vi "NewRobotTurningAroundBall.vi"(6 "Target":dbl[](array[numeric]), 7 "Game":refnum<class "Game.lvclass">, 8 "error in (no error)":errorcluster, 9 "Raio":dbl=123.0, 10 "Robot in":refnum<class "Robot.lvclass">, 11 "KickToSkill in":refnum<class "KickToSkill.lvclass">) -> (0 "error out":errorcluster, 1 "Robot out":refnum<class "Robot.lvclass">, 3 "KickToSkill out":refnum<class "KickToSkill.lvclass">)   [LabVIEW 2021, in "KickToSkill.lvclass"]
uses:
  KickToSkill.lvclass
  robotTurningBallStates.ctl
  <vilib>/Analysis/NI_AALPro.lvlib
  <vilib>/Analysis/coordinate.llb/2D Cartesian Coordinate Rotation (Scalar).vi
  Game_class/Game.lvclass
  Robot_class/Robot.lvclass
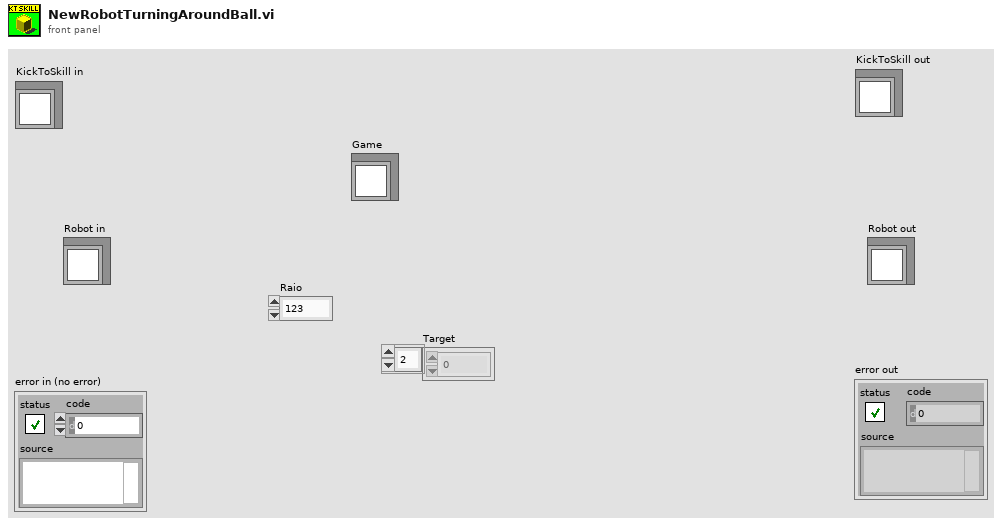
[diagram p1: front panel]
types:
  T1 = typedef "KickToSkill.lvclass/robotTurningBallStates.ctl" = enum16{"go straight to the target", "go to point A", "circulating the ball", "lining up", "shoot"}
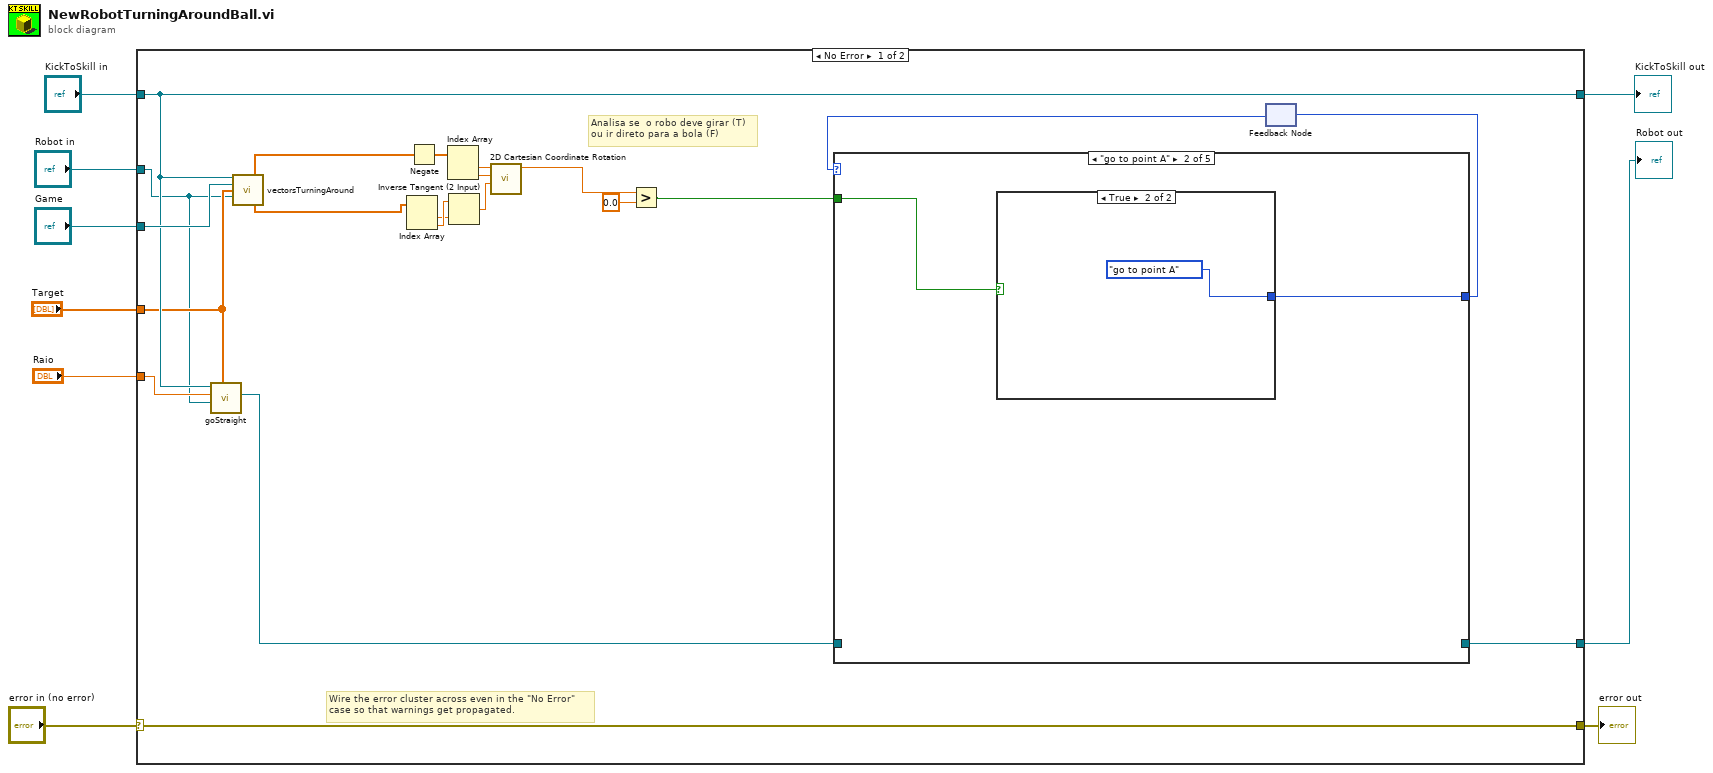
[diagram p0: block diagram]
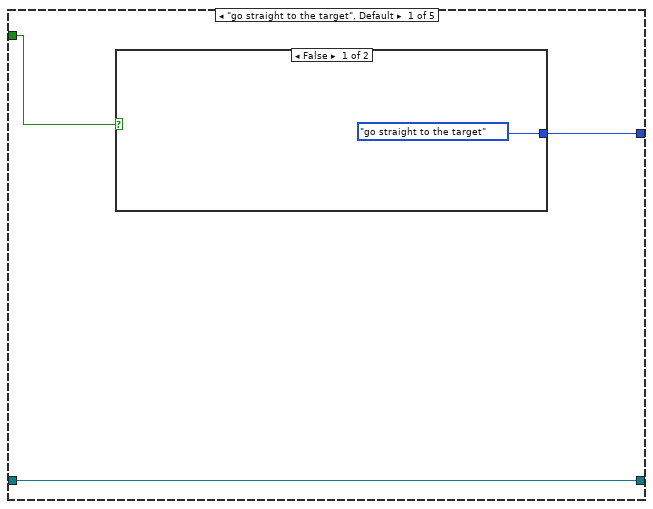
[diagram p2: hidden frame]
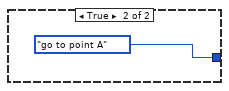
[diagram p3: hidden frame]
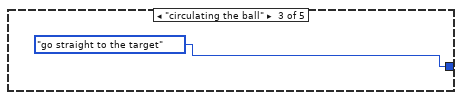
[diagram p5: hidden frame]
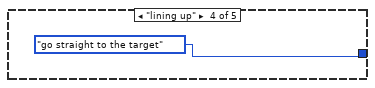
[diagram p6: hidden frame]
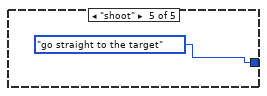
[diagram p7: hidden frame]
diagram:
  n1 = case shown="No Error" "error in (no error)" {
    selector: "error in (no error)" -> [w30 w44]
    tunnel: [w30 w44] -> w8
    tunnel: [w15 w43] -> w6
    tunnel: "KickToSkill in" -> [w15 w43]
    tunnel: "Robot in" -> [w12 w42]
    tunnel: "Target" -> [w14 _]
    tunnel: "Game" -> [w29 _]
    tunnel: "Raio" -> [w13 _]
    tunnel: [w10 w42] -> w1
    frame No Error {
      # "Analisa se  o robo deve girar (T)\nou ir direto para a bola (F)"
      # "Wire the error cluster across even in the \"No Error\"\ncase so that warnings get propagated."
      n2 = call "goStraight.vi"("Target"=w14, "Robot in"=w12, "Raio"=w13, "KickToSkill in"=w15) -> ("Robot out"=w11:refnum<class "Robot.lvclass">)  [unwired: 5 in, 2 out]
      n3 = call "vectorsTurningAround.vi"("KickToSkill in"=w15, "Game"=w29, "Target"=w14, "Robot in"=w12) -> ("Ball - Target"=w20:dbl[], "Robot - Ball"=w19:dbl[])  [unwired: 4 in, 6 out]
      n4 = Index Array(array=w19) -> (element #1=w23:dbl, element #2=w24:dbl)  [unwired: 2 in]
      n5 = Negate(x=w20) -> (-x=w21:dbl[])
      n6 = Index Array(array=w21) -> (element #1=w25:dbl, element #2=w26:dbl)  [unwired: 2 in]
      n7 = Inverse Tangent (2 Input)(1:w23, 2:w24) -> (0:w22:dbl)
      n8 = call-poly <vilib>:"2D Cartesian Coordinate Rotation.vi"("theta"=w22, "y"=w26, "x"=w25) -> ("x out"=w18:dbl)  [unwired: 6 in, 2 out]
      n9 = Greater?(x=w18, y=0.0) -> (0:w16:bool)
      n10 = feedback #1() -> (w27:T1)  [unwired: 1 in]
      n11 = case shown="\"go to point A\"" w27 {
        tunnel: [w33 w37 robotTurningBallStates."go straight to the target" ("Enum") robotTurningBallStates."go straight to the target" ("Enum") robotTurningBallStates."go straight to the target" ("Enum")] -> w28
        tunnel: w16 -> [w32 w36 _ _ _]
        tunnel: w11 -> [w31 _ _ _ _]
        tunnel: [w31 _ _ _ _] -> w10
        frame "go straight to the target", Default {
          n12 = case shown="False" w32 {
            tunnel: [robotTurningBallStates."go straight to the target" ("Enum") robotTurningBallStates."go to point A" ("Enum")] -> w33
            frame False {
            }
            frame True {
            }
          }
        }
        frame "go to point A" {
          n13 = case shown="True" w36 {
            tunnel: [_ robotTurningBallStates."go to point A" ("Enum")] -> w37
            frame False {
            }
            frame True {
            }
          }
        }
        frame "circulating the ball" {
        }
        frame "lining up" {
        }
        frame "shoot" {
        }
      }
      n14 = feedback-in #1(w28) -> ()
    }
    frame Error {
    }
  }
  "error out" <- w8
  "KickToSkill out" <- w6
  "Robot out" <- w1
